vi "webot.vi"() -> ()   [LabVIEW 2015]
uses:
  G_NAV.vi
  G_VEH.vi
panel:
  out "error out 2":errorcluster
  out "error out":errorcluster
  out "data":sgl[](array[numeric])
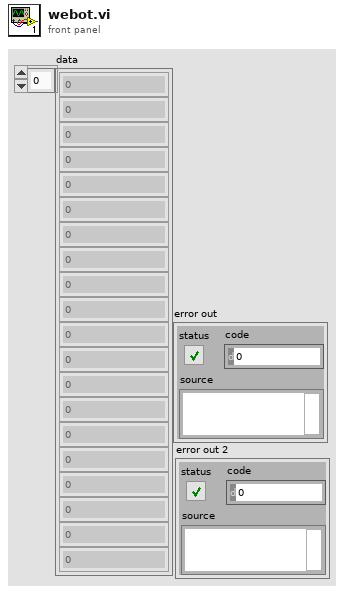
[diagram p1: front panel]
types:
  T1 = enum16{"big-endian, network order", "native, host order", "little-endian"}
  T2 = cluster{"sop1":u8, "sop2":u8, "sop3":u8, "header_length":u8, "number":u16, "type":u8, "port_address":u8, "length":u16, "sequence":u16, "idle":u8, "gps_stat":u8, "gps_week":u16, "millisecs":u32, "status":u32, "crc":u16, "version":u16}
  T3 = cluster{"GPSTime":dbl, "accel[0]":sgl, "accel[1]":sgl, "accel[2]":sgl, "pqr[0]":sgl, "pqr[1]":sgl, "pqr[2]":sgl, "llh[0]":dbl, "llh[1]":dbl, "llh[2]":dbl, "vel_ned[0]":sgl, "vel_ned[1]":sgl, "vel_ned[2]":sgl, "attitude[0]":sgl, "attitude[1]":sgl, "attitude[2]":sgl, "vel_bxyz[0]":sgl, "vel_bxyz[1]":sgl, "vel_bxyz[2]":sgl, "lcc[0]":sgl, "lcc[1]":sgl, "lcc[2]":sgl, "CovKalman[0]":sgl, "CovKalman[1]":sgl, "CovKalman[2]":sgl, "CovKalman[3]":sgl, "CovKalman[4]":sgl, "CovKalman[5]":sgl, "llh_GPS[0]":sgl, "llh_GPS[1]":sgl, "llh_GPS[2]":sgl, "vel_GPS[0]":sgl, "vel_GPS[1]":sgl, "vel_GPS[2]":sgl, "heading_Magnetic":sgl, "heading_GPS":sgl, "GPSStatus":u16, "FailureCode":u16, "DataChecksum":u16}
  T4 = cluster{"sol_stat":u32, "pos_type":u32, "lat":dbl, "lon":dbl, "hgt":dbl, "und":sgl, "datum_id":i32, "latdev":sgl, "londev":sgl, "hgtdev":sgl, "ref_station_id 0":i8, "ref_station_id 1":i8, "ref_station_id 2":i8, "ref_station_id 3":i8, "lag":sgl, "age":sgl, "sats":u8, "gps_l1_ranges":u8, "gps_l1_mask_ranges":u8, "gps_l2_mask_ranges":u8, "reserved":i8, "ext_sol_stat":u8, "reserved2":u8, "sig_mask":u8}
  T5 = cluster{"Steer_input":dbl, "Steer_output":dbl, "VS_des":dbl, "VS_can":dbl, "heading":dbl, "auto":bool, "run":bool, "x":dbl, "y":dbl}
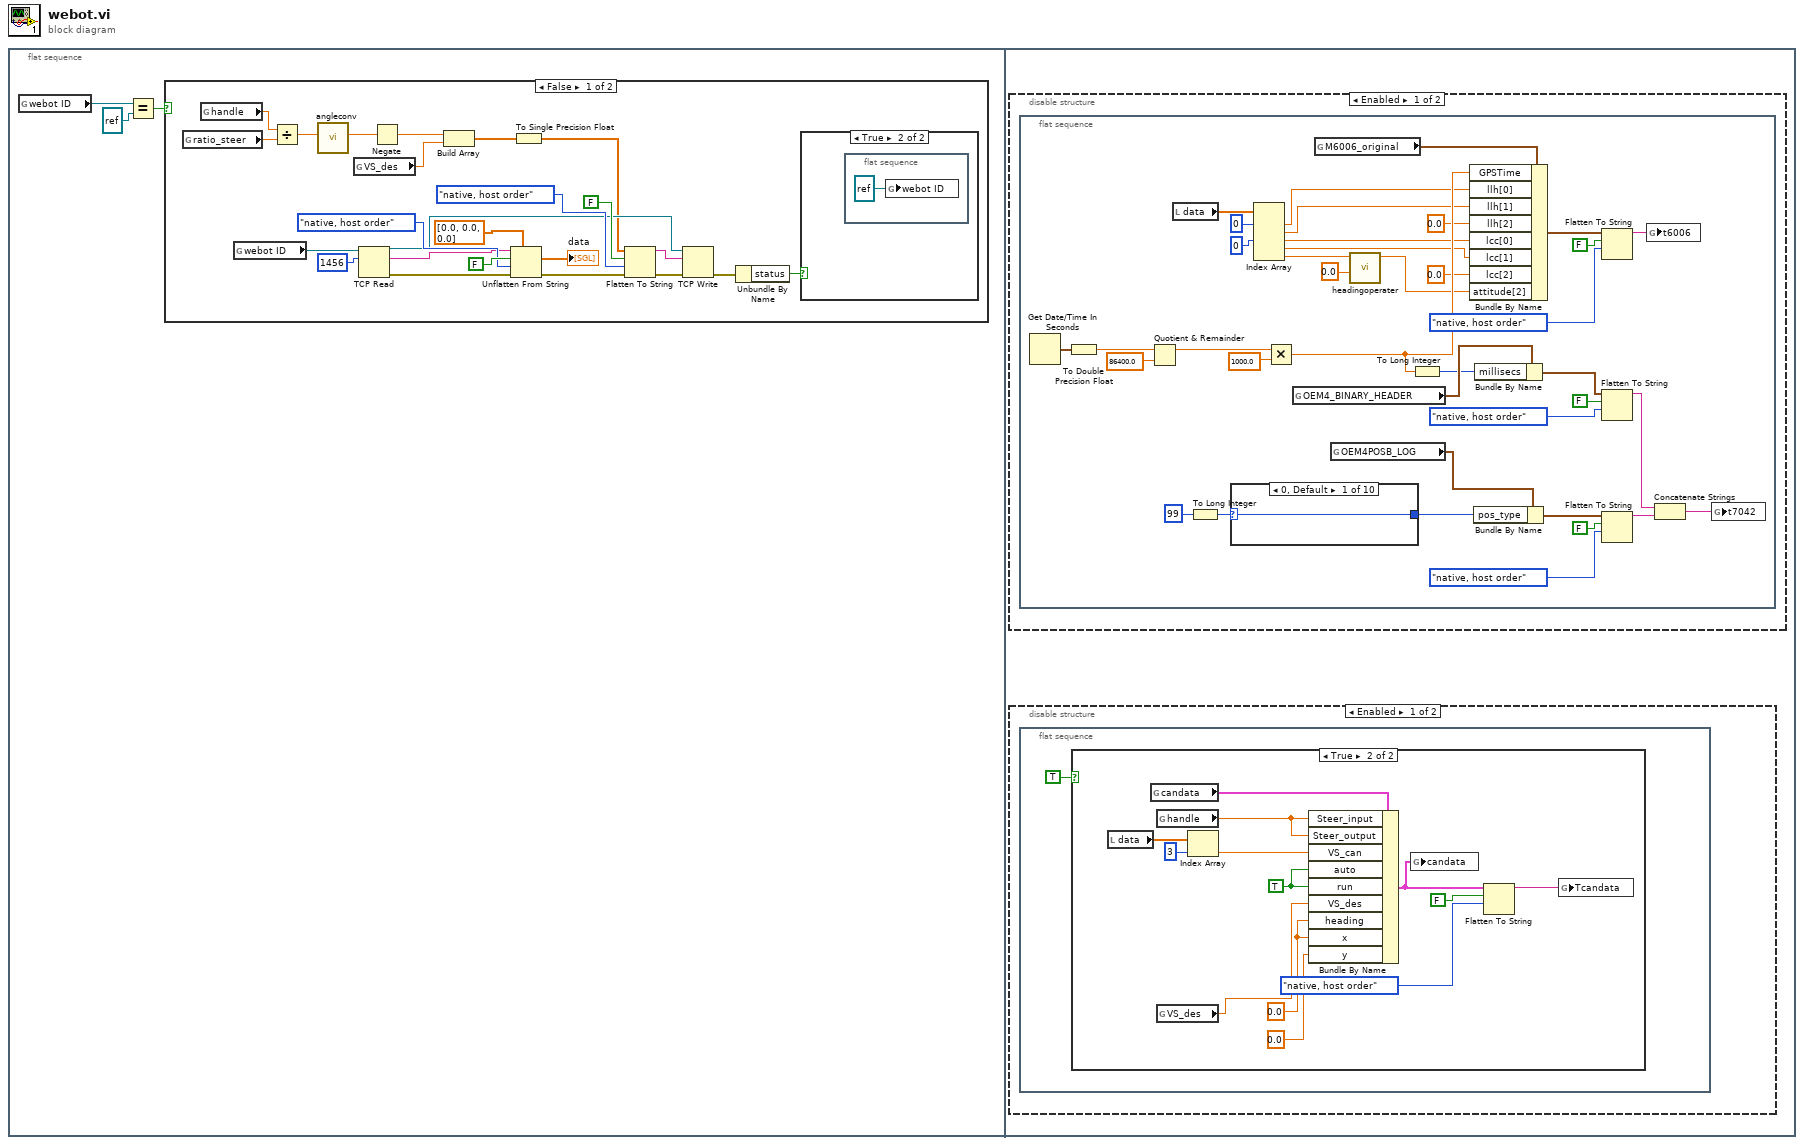
[diagram p0: block diagram]
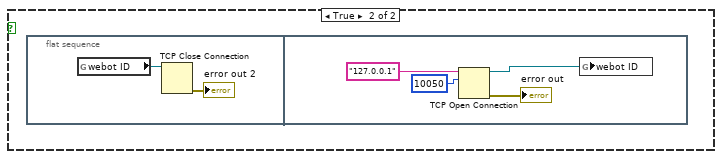
[diagram p3: hidden frame]
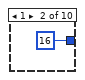
[diagram p6: hidden frame]
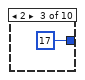
[diagram p7: hidden frame]
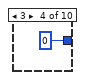
[diagram p8: hidden frame]
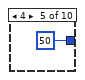
[diagram p9: hidden frame]
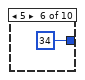
[diagram p10: hidden frame]
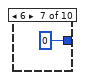
[diagram p11: hidden frame]
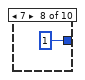
[diagram p12: hidden frame]
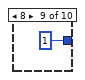
[diagram p13: hidden frame]
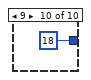
[diagram p14: hidden frame]
diagram:
  n1 = flat-sequence {
    frame #0 {
      n2 = global read "G_NAV.vi" "webot ID"() -> (w3:refnum<k5>)
      n3 = Equal?(x=w3, y=refnum<k5> refnum ("connection ID")) -> (x = y?=w1:bool)
      n4 = case shown="False" w1 {
        frame False {
          n5 = global read "G_VEH.vi" "ratio_steer"() -> (w11:dbl)
          n6 = global read "G_VEH.vi" "handle"() -> (w12:dbl)
          n7 = global read "G_NAV.vi" "webot ID"() -> (w14:refnum<k5>)
          n8 = Divide(x=w12, y=w11) -> (x/y=w8:dbl)
          n9 = call "angleconv.vi"("deg"=w8) -> ("rad"=w5:dbl)  [unwired: 9 in, 1 out]
          n10 = global read "G_VEH.vi" "VS_des"() -> (w13:dbl)
          n11 = TCP Read(connection ID=w14, bytes to read=1456) -> (connection ID out=w18:refnum<k5>, data out=w16:string, error out=w17:errorcluster)  [unwired: 1 in, 2 out]
          n12 = Negate(x=w5) -> (-x=w4:dbl)
          n13 = Build Array(w4, w13) -> (w7:dbl[])
          n14 = Unflatten From String(type=sgl[] [0.0, 0.0, 0.0] ("data"), binary string=w16, data includes array or string size? (T)=FALSE, byte order (0:big-endian, network order)=T1."native, host order", error in (no error)=w17) -> (value=→"data":sgl[], error out=w26:errorcluster)  [unwired: 1 out]
          n15 = To Single Precision Float(number=w7) -> (single precision float=w6:sgl[])
          n16 = Flatten To String(anything=w6, prepend array or string size? (T)=FALSE, byte order (0:big-endian, network order)=T1."native, host order", error in (no error)=w26) -> (data string=w25:string, error out=w27:errorcluster)  [unwired: 1 out]
          n17 = TCP Write(connection ID=w18, data in=w25, error in (no error)=w27) -> (error out=w10:errorcluster)  [unwired: 1 in, 2 out]
          n18 = Unbundle By Name(w10) -> ("status"=w9:bool)
          n19 = case shown="True" w9 {
            frame False {
            }
            frame True {
              n20 = flat-sequence {
                frame #0 {
                  n21 = global write "G_NAV.vi" "webot ID"(refnum<k5> refnum ("connection ID")) -> ()
                }
              }
            }
          }
        }
        frame True {
          n22 = flat-sequence {
            frame #0 {
              n23 = global read "G_NAV.vi" "webot ID"() -> (w30:refnum<k5>)
              n24 = TCP Close Connection(connection ID=w30) -> (error out=→"error out 2":errorcluster)  [unwired: 2 in, 1 out]
            }
            frame #1 {
              n25 = TCP Open Connection(address="127.0.0.1", remote port or service name=u16 10050) -> (connection ID=w34:refnum<k5>, error out=→"error out":errorcluster)  [unwired: 1 in, 2 out]
              n26 = global write "G_NAV.vi" "webot ID"(w34) -> ()
            }
          }
        }
      }
    }
    frame #1 {
      n27 = disable-structure shown="Enabled" {
        frame Enabled {
          n28 = flat-sequence {
            frame #0 {
              n29 = Get Date/Time In Seconds() -> (seconds since 1Jan1904=w68:timestamp)
              n30 = To Double Precision Float(number=w68) -> (double precision float=w64:dbl)
              n31 = Quotient & Remainder(x=w64, y=86400.0) -> (x-y*floor(x/y)=w66:dbl)  [unwired: 1 out]
              n32 = local read "data"() -> (w61:sgl[])
              n33 = To Long Integer(number=99) -> (32bit integer=w84:i32)
              n34 = case shown="0, Default" w84 {
                selector: w84 -> [w87 _ _ _ _ _ _ _ _ _]
                tunnel: [w87 16 17 0 50 34 0 1 1 18] -> w83
                frame 0, Default {
                }
                frame 1 {
                }
                frame 2 {
                }
                frame 3 {
                }
                frame 4 {
                }
                frame 5 {
                }
                frame 6 {
                }
                frame 7 {
                }
                frame 8 {
                }
                frame 9 {
                }
              }
              n35 = Index Array(array=w61, index #1=0 ("index"), index #3=0 ("index")) -> (element #1=w59:sgl, element #2=w58:sgl, element #3=w57:sgl, element #4=w55:sgl, element #5=w51:sgl)  [unwired: 3 in]
              n36 = Multiply(x=w66, y=1000.0) -> (x*y=w62:dbl)
              n37 = global read "G_NAV.vi" "OEM4_BINARY_HEADER"() -> (w82:T2)
              n38 = global read "G_NAV.vi" "M6006_original"() -> (w86:T3)
              n39 = global read "G_NAV.vi" "OEM4POSB_LOG"() -> (w85:T4)
              n40 = call "headingoperater.vi"("h1"=0.0, "h2"=w51) -> ("h2+h1"=w49:dbl)  [unwired: 8 in, 1 out]
              n41 = To Long Integer(number=w62) -> (32bit integer=w63:i32)
              n42 = Bundle By Name(cluster=w86, "GPSTime"=w62, "llh[0]"=w59, "llh[1]"=w58, "llh[2]"=0.0, "lcc[0]"=w57, "lcc[1]"=w55, "lcc[2]"=sgl 0.0, "attitude[2]"=w49) -> (w81:T3)
              n43 = Bundle By Name(cluster=w85, "pos_type"=w83) -> (w72:T4)
              n44 = Bundle By Name(cluster=w82, "millisecs"=w63) -> (w76:T2)
              n45 = Flatten To String(anything=w81, prepend array or string size? (T)=FALSE, byte order (0:big-endian, network order)=T1."native, host order") -> (data string=w78:string)  [unwired: 1 in, 2 out]
              n46 = Flatten To String(anything=w76, prepend array or string size? (T)=FALSE, byte order (0:big-endian, network order)=T1."native, host order") -> (data string=w71:string)  [unwired: 1 in, 2 out]
              n47 = Flatten To String(anything=w72, prepend array or string size? (T)=FALSE, byte order (0:big-endian, network order)=T1."native, host order") -> (data string=w70:string)  [unwired: 1 in, 2 out]
              n48 = global write "G_NAV.vi" "t6006"(w78) -> ()
              n49 = Concatenate Strings(w71, w70) -> (w69:string)
              n50 = global write "G_NAV.vi" "t7042"(w69) -> ()
            }
          }
        }
        frame Disabled {
        }
      }
      n51 = disable-structure shown="Enabled" {
        frame Enabled {
          n52 = flat-sequence {
            frame #0 {
              n53 = case shown="True" TRUE {
                frame False {
                }
                frame True {
                  w40 = TRUE ("auto")
                  w41 = 0.0 ("x")
                  n54 = local read "data"() -> (w38:sgl[])
                  n55 = global read "G_VEH.vi" "candata"() -> (w44:T5)
                  n56 = global read "G_VEH.vi" "handle"() -> (w36:dbl)
                  n57 = global read "G_VEH.vi" "VS_des"() -> (w43:dbl)
                  n58 = Index Array(array=w38, index=3) -> (element=w37:sgl)
                  n59 = Bundle By Name(cluster=w44, "Steer_input"=w36, "Steer_output"=w36, "VS_can"=w37, "auto"=w40, "run"=w40, "VS_des"=w43, "heading"=w41, "x"=w41, "y"=0.0) -> (w48:T5)
                  n60 = global write "G_VEH.vi" "candata"(w48) -> ()
                  n61 = Flatten To String(anything=w48, prepend array or string size? (T)=FALSE, byte order (0:big-endian, network order)=T1."native, host order") -> (data string=w45:string)  [unwired: 1 in, 2 out]
                  n62 = global write "G_VEH.vi" "Tcandata"(w45) -> ()
                }
              }
            }
          }
        }
        frame Disabled {
        }
      }
    }
  }
